vi "SyncLoop.vi"(8 "error in (no error)":errorcluster, 11 "Local in":refnum<class "Local.lvclass">) -> (0 "error out":errorcluster, 1 "Lock":bool, 2 "Time Ref Offset (ns)":dbl format="%#_12f", 3 "Local out":refnum<class "Local.lvclass">, 4 "LostLock":bool, 6 "ObtainLock":bool)   [LabVIEW 2014, in "SyncPlugins.lvlib" / "Local.lvclass"]
uses:
  Local.lvclass
  SyncPluginBase/SyncPluginBase.lvclass/SyncPluginBase.ctl
  SyncPluginBase/Accessors/Write Locked.vi
  SyncPluginBase/Accessors/Write Run.vi
  SyncPluginBase/Accessors/Write PPSTime.vi
  SyncPluginBase/Accessors/Read Locked.vi
panel:
  out "time stamp out":timestamp format="%^<%.3X\n%x>T"
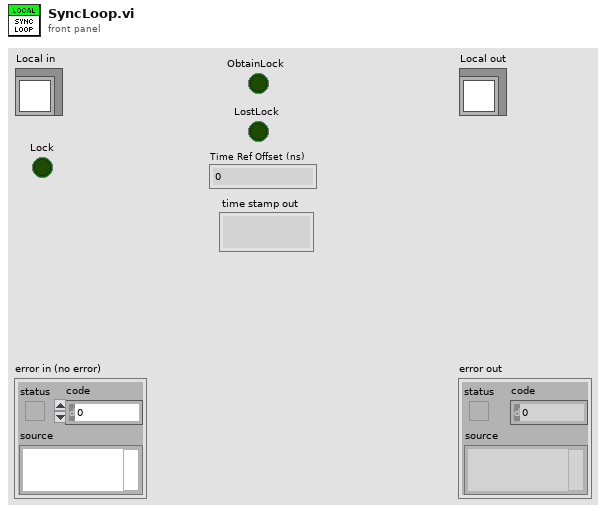
[diagram p1: front panel]
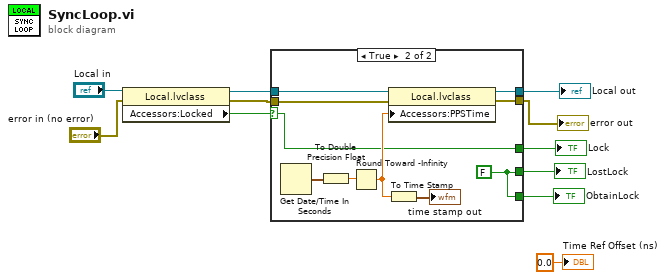
[diagram p0: block diagram]
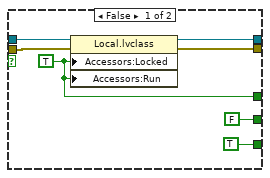
[diagram p2: hidden frame]
diagram:
  n1 = property class="Local.lvclass"(reference="Local in", error in="error in (no error)") -> (reference out=w9:refnum<class "Local.lvclass">, error out=w3:errorcluster, "Accessors:Locked"=w10:bool)
  n2 = case shown="True" w10 {
    selector: w10 -> [_ w19]
    tunnel: w9 -> [w18 w27]
    tunnel: [TRUE w28] -> w8
    tunnel: [FALSE w28] -> w7
    tunnel: [w15 w26] -> w6
    tunnel: w3 -> [w14 w22]
    tunnel: [w13 w21] -> w2
    tunnel: [w12 w19] -> w1
    frame False {
      w12 = TRUE ("Locked")
      n3 = property class="Local.lvclass"(reference=w18, error in=w14, "Accessors:Locked"=w12, "Accessors:Run"=w12) -> (reference out=w15:refnum<class "Local.lvclass">, error out=w13:errorcluster)
    }
    frame True {
      w28 = FALSE
      n4 = Get Date/Time In Seconds() -> (seconds since 1Jan1904=w25:timestamp)
      n5 = To Double Precision Float(number=w25) -> (double precision float=w24:dbl)
      n6 = Round Toward -Infinity(1:w24) -> (0:w20:dbl)
      n7 = property class="Local.lvclass"(reference=w27, error in=w22, "Accessors:PPSTime"=w20) -> (reference out=w26:refnum<class "Local.lvclass">, error out=w21:errorcluster)
      n8 = To Time Stamp(1:w20) -> (0:→"time stamp out":timestamp)
    }
  }
  "error out" <- w2
  "Local out" <- w6
  "ObtainLock" <- w8
  "LostLock" <- w7
  "Lock" <- w1
  "Time Ref Offset (ns)" <- 0.0 ("Time Ref Offset (ns)")
